vi "oauth2-pkce.vi"(8 "error in (no error)":errorcluster, 9 "code_verifier":string, 10 "client_id":string, 11 "authorization_code":string) -> (0 "error out":errorcluster, 3 "access_token":string)   [LabVIEW 2015, in "lv-dropbox.lvlib"]
uses:
  lv-dropbox.lvlib
  private/_controls/content_type.ctl
  <vilib>/httpClient/POSTBuffer.vi
  <vilib>/httpClient/LabVIEWHTTPClient.lvlib
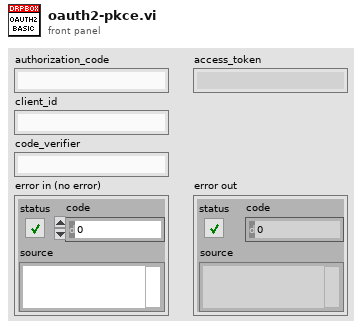
[diagram p1: front panel]
types:
  T1 = typedef "lv-dropbox.lvlib/content_type.ctl" = enum16{"<content_type>", "application/json", "application/octet-stream", "application/x-www-form-urlencoded"}
  T2 = cluster{"access_token":string, "expires_in":dbl, "token_type":string}
  T3 = typedef "LabVIEWHTTPClient.lvlib/ClientHandle.ctl" = refnum<k1>
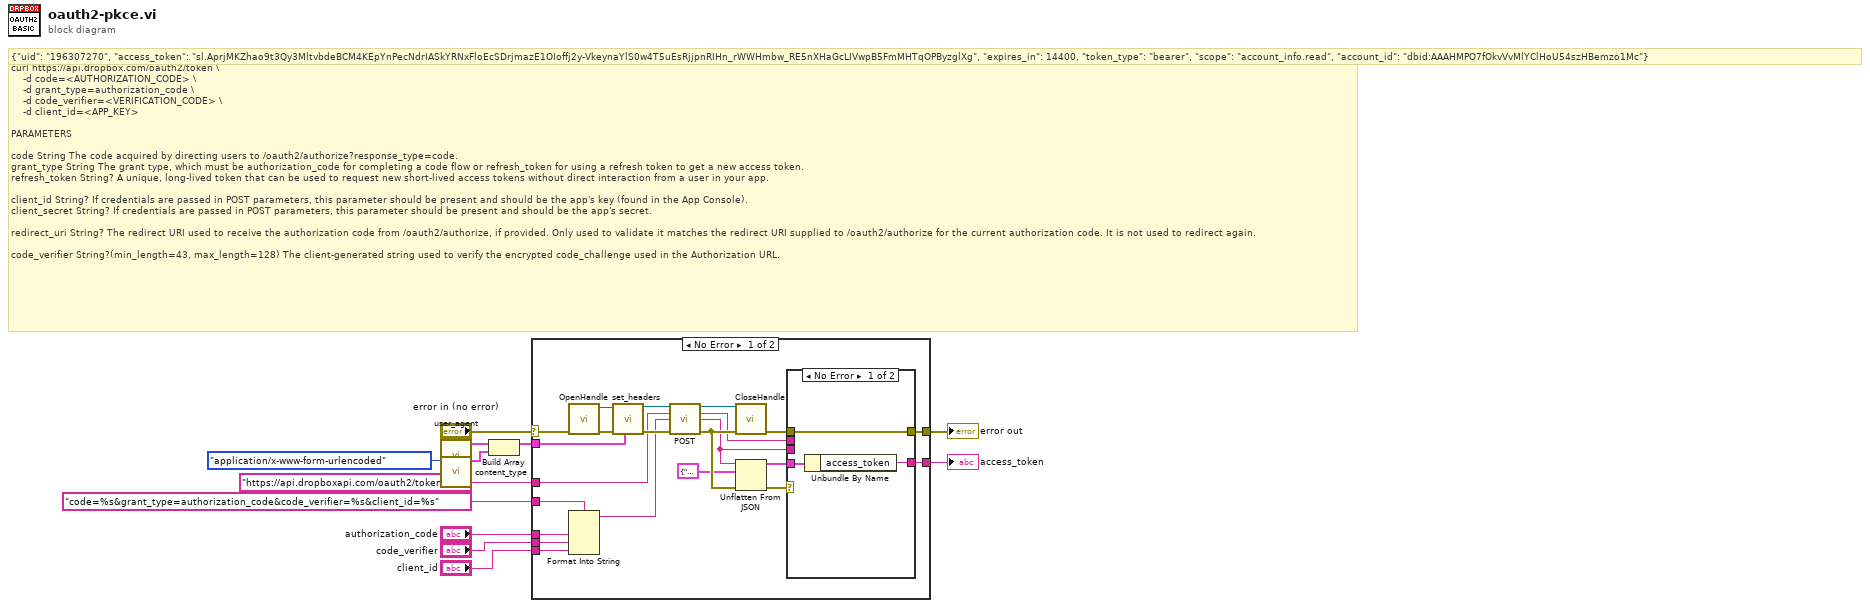
[diagram p0: block diagram]
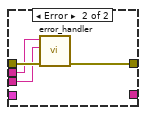
[diagram p2: hidden frame]
diagram:
  # "{\"uid\": \"196307270\", \"access_token\": \"sl.AprjMKZhao9t3Qy3MltvbdeBCM4KEpYnPecNdrIASkYRNxFloEcSDrjmazE1OIoffj2y-VkeynaYlS0w4T5uEsRjjpnRIHn_rWWHmbw_RE5nXHaGcLIVwpB5FmMHTqOPByzglXg\", \"expires_in\": 14400, \"token_type\": \"bearer\", \"scope\": \"account_info.read\", \"account_id\": \"dbid:AAAHMPO7fOkvVvMlYClHoU54szHBemzo1Mc\"}"
  # "curl https://api.dropbox.com/oauth2/token \\\n    -d code=<AUTHORIZATION_CODE> \\\n    -d grant_type=authorization_code \\\n    -d code_verifier=<VERIFICATION_CODE> \\\n    -d client_id=<APP_KEY>\n\nPARAMETERS\n\ncode String The code acquired by directing users to /oauth2/authorize?response_type=code.\ngrant_type String The grant type, which must be authorization_code for completing a code flow or refresh_token for using a refresh token to get a new access token.\nrefresh_token String? A unique, long-lived token that can be used to request new short-lived access tokens without direct interaction from a user in your app.\n\nclient_id String? If credentials are passed in POST parameters, this parameter should be present and should be the app's key (found in the App Console).\nclient_secret String? If credentials are passed in POST parameters, this parameter should be present and should be the app's secret.\n\nredirect_uri String? The redirect URI used to receive the authorization code from /oauth2/authorize, if provided. Only used to validate it matches the redirect URI supplied to /oauth2/authorize for the current authorization code. It is not used to redirect again.\n\ncode_verifier String?(min_length=43, max_length=128) The client-generated string used to verify the encrypted code_challenge used in the Authorization URL."
  n1 = call "user_agent.vi"() -> ("header"=w8:cluster{"header":string, "value":string})  [unwired: 11 in]
  n2 = call "content_type.vi"("content_type"=content_type."application/x-www-form-urlencoded") -> ("header"=w11:cluster{"header":string, "value":string})  [unwired: 10 in]
  n3 = Build Array(w8, w11) -> (w7:cluster{"header":string, "value":string}[])
  n4 = case shown="No Error" "error in (no error)" {
    selector: "error in (no error)" -> [w28 w42]
    tunnel: "https://api.dropboxapi.com/oauth2/token" ("url") -> [w32 _]
    tunnel: w7 -> [w26 _]
    tunnel: [w21 w42] -> w9
    tunnel: "code=%s&grant_type=authorization_code&code_verifier=%s&client_id=%s" -> [w18 _]
    tunnel: "code_verifier" -> [w17 _]
    tunnel: "authorization_code" -> [w15 _]
    tunnel: "client_id" -> [w14 _]
    tunnel: [w13 _] -> w1
    frame No Error {
      n5 = call <vilib>:"OpenHandle.vi"("error in (no error)"=w28) -> ("client handle out"=w29:T3, "error out"=w27:errorcluster)  [unwired: 13 in]
      n6 = Format Into String(format string=w18, w15, w17, w14) -> (resulting string=w16:string)  [unwired: 2 in, 1 out]
      n7 = call "set_headers.vi"("header_value []"=w26, "error in (no error)"=w27, "client_handle in"=w29) -> ("error out"=w33:errorcluster, "client_handle out"=w25:T3)  [unwired: 7 in]
      n8 = call-poly <vilib>:"POST.vi"("client handle"=w25, "url"=w32, "buffer"=w16, "error in (no error)"=w33) -> ("client handle out"=w24:T3, "headers"=w20:string, "body"=w19:string, "error out"=w34:errorcluster)  [unwired: 8 in]
      n9 = call <vilib>:"CloseHandle.vi"("client handle"=w24, "error in (no error)"=w34) -> ("error out"=w22:errorcluster)  [unwired: 13 in]
      n10 = Unflatten From JSON(JSON string=w19, type and defaults=T2 {"access_token"="", "expires_in"=0.0, "token_type"=""} ("value"), error in (no error)=w34) -> (value=w30:T2, error out=w23:errorcluster)  [unwired: 4 in]
      n11 = case shown="No Error" w23 {
        tunnel: w30 -> [w36 _]
        tunnel: w22 -> [w37 w41]
        tunnel: [w37 w38] -> w21
        tunnel: w20 -> [_ w40]
        tunnel: w19 -> [_ w39]
        tunnel: [w35 _] -> w13
        frame No Error {
          n12 = Unbundle By Name(w36) -> ("access_token"=w35:string)
        }
        frame Error {
          n13 = call "error_handler.vi"("error in (no error)"=w41, "body"=w39, "headers"=w40) -> ("error out"=w38:errorcluster)  [unwired: 8 in]
        }
      }
    }
    frame Error {
    }
  }
  "error out" <- w9
  "access_token" <- w1
